vi "E21_UART.vi"() -> ()   [LabVIEW 2026]
uses:
  <vilib>/Instr/_visa.llb/VISA Configure Serial Port (Instr).vi
  <vilib>/ptbypt/NI_PtbyPt.lvlib
panel:
  out "error out":errorcluster
  out "Histeresis":bool
  out "Alarma":bool
  in  "Umbral minimo":dbl
  in  "Umbral maximo":dbl
  in  "Excel":bool
  in  "Filtro EMA":bool
  out "Waveform Chart":dbl(graph)
  in  "Datos a enviar":string
  out "Dato recibido":string
  in  "VISA resource name":refnum<visa-resource-name>
  in  "data bits (8)":u16=8 min=5 max=8 step=1
  in  "baud rate (9600)":u32=9600
  in  "Lectura":bool
  in  "Escritura":bool
  in  "stop":bool
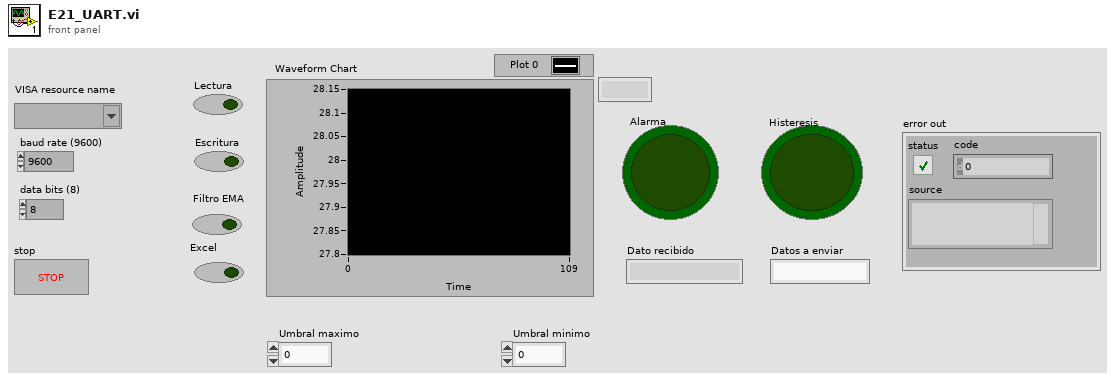
[diagram p1: front panel]
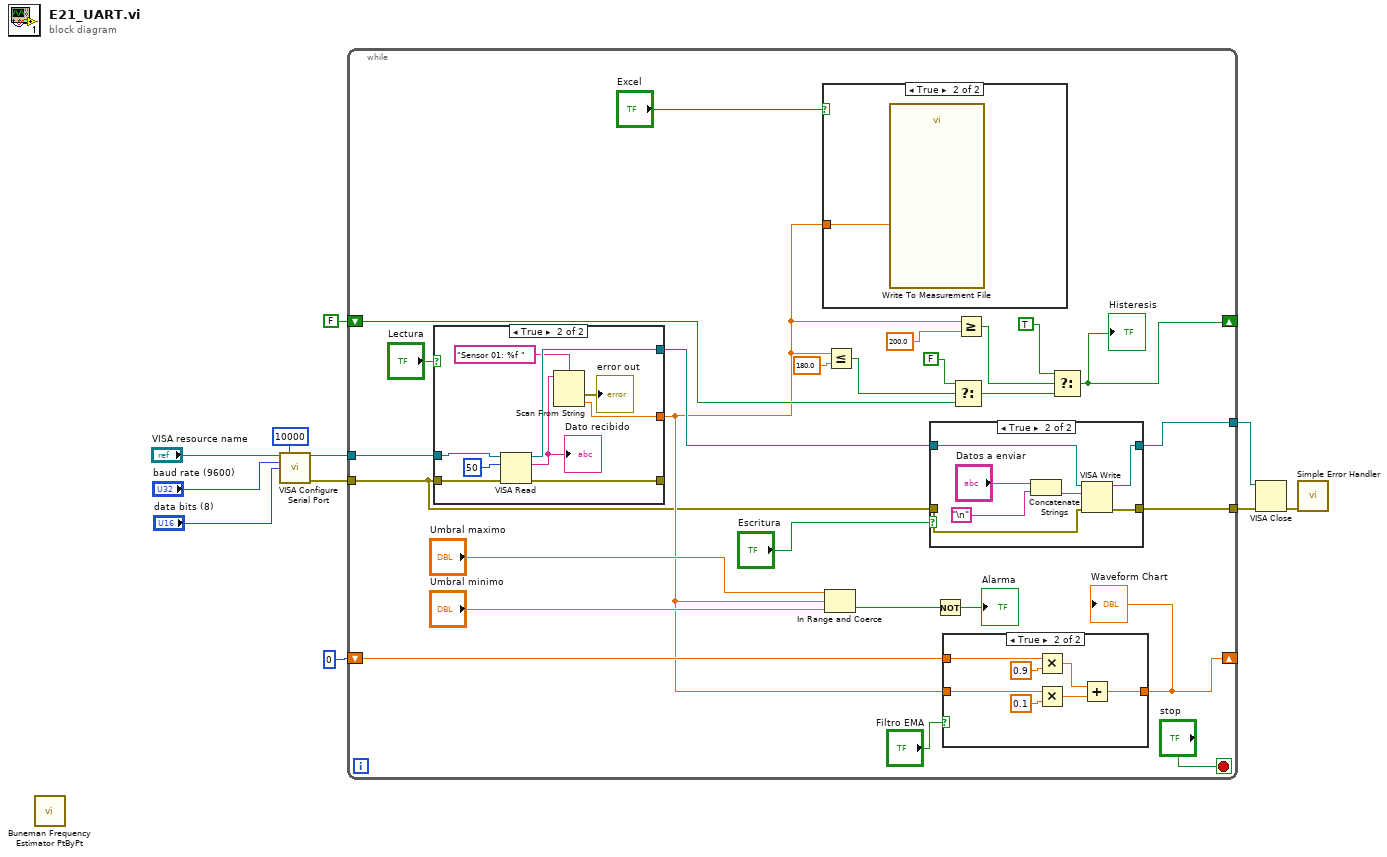
[diagram p0: block diagram]
diagram:
  n1 = call <vilib>:"Buneman Frequency Estimator PtByPt.vi"() -> ()  [unwired: 4 in, 2 out]
  n2 = call-poly "VISA Configure Serial Port"("VISA resource name"="VISA resource name", "timeout (10sec)"=u32 10000, "baud rate (9600)"="baud rate (9600)", "data bits (8)"="data bits (8)") -> ("VISA resource name out"=w11:refnum<visa-resource-name>, "error out"=w7:errorcluster)  [unwired: 10 in]
  n3 = while {
    tunnel: w11 -> [w34]
    tunnel: w7 -> [w12]
    tunnel: [w32] -> w5
    tunnel: [w31] -> w6
    shift-right: [w24] -> _
    shift-left: 0 -> [w23]
    shift-right: [w14] -> _
    shift-left: FALSE -> [w16]
    stop <- "stop" stop-if-true
    n4 = case shown="True" "Lectura" {
      tunnel: w34 -> [w57 w66]
      tunnel: w12 -> [w56 w64]
      tunnel: [w56 w63] -> _
      tunnel: [w57 w62] -> w33
      tunnel: [_ w60] -> w13
      frame False {
      }
      frame True {
        n5 = VISA Read(VISA resource name=w66, byte count=u32 50, error in (no error)=w64) -> (VISA resource name out=w62:refnum<visa-resource-name>, read buffer=w61:string, error out=w63:errorcluster)  [unwired: 1 out]
        "Dato recibido" <- w61
        n6 = Scan From String(format string="Sensor 01: %f ", input string=w61) -> (error out=→"error out":errorcluster, output 1=w60:dbl)  [unwired: 3 in, 2 out]
      }
    }
    n7 = case shown="True" "Excel" {
      tunnel: w13 -> [_ w38]
      frame False {
      }
      frame True {
        n8 = call "Write To Measurement File"("Signals"=w38) -> ()  [unwired: 16 in, 3 out]
      }
    }
    n9 = In Range and Coerce(upper limit="Umbral maximo", x=w13, lower limit="Umbral minimo") -> (In Range?=w26:bool)  [unwired: 1 out]
    n10 = Less Or Equal?(x=w13, y=180.0) -> (x <= y?=w22:bool)
    n11 = case shown="True" "Escritura" {
      tunnel: w12 -> [w47 w55]
      tunnel: [w47 w54] -> w32
      tunnel: w33 -> [w48 w53]
      tunnel: [w48 w52] -> w31
      frame False {
      }
      frame True {
        n12 = Concatenate Strings("Datos a enviar", "\n") -> (w49:string)
        n13 = VISA Write(VISA resource name=w53, write buffer=w49, error in (no error)=w55) -> (VISA resource name out=w52:refnum<visa-resource-name>, error out=w54:errorcluster)  [unwired: 1 out]
      }
    }
    n14 = Not(x=w26) -> (.not. x?=→"Alarma":bool)
    n15 = case shown="True" "Filtro EMA" {
      tunnel: w13 -> [w39 w46]
      tunnel: w23 -> [_ w44]
      tunnel: [w39 w40] -> w24
      frame False {
      }
      frame True {
        n16 = Multiply(x=w44, y=0.9) -> (x*y=w41:dbl)
        n17 = Multiply(x=w46, y=0.1) -> (x*y=w42:dbl)
        n18 = Add(x=w41, y=w42) -> (x+y=w40:dbl)
      }
    }
    "Waveform Chart" <- w24
    n19 = Select(t=FALSE, s=w22, f=w16) -> (s? t:f=w15:bool)
    n20 = Greater Or Equal?(x=w13, y=200.0) -> (x >= y?=w21:bool)
    n21 = Select(t=TRUE, s=w21, f=w15) -> (s? t:f=w14:bool)
    "Histeresis" <- w14
  }
  n22 = VISA Close(VISA resource name=w6, error in (no error)=w5) -> (error out=w4:errorcluster)
  n23 = call <vilib>:"Simple Error Handler.vi"("error in (no error)"=w4) -> ()  [unwired: 4 in, 5 out]
